vi "quote and escape json string 2.vi"(11 "base string":string) -> (3 "String out":string)   [LabVIEW 2020, in "JSONtext.lvlib"]
uses:
  <vilib>/JDP Science/JSONtext/JSONtext.lvlib
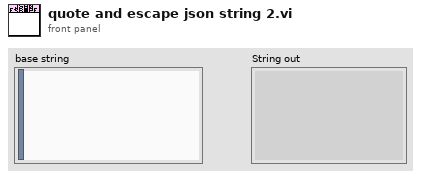
[diagram p1: front panel]
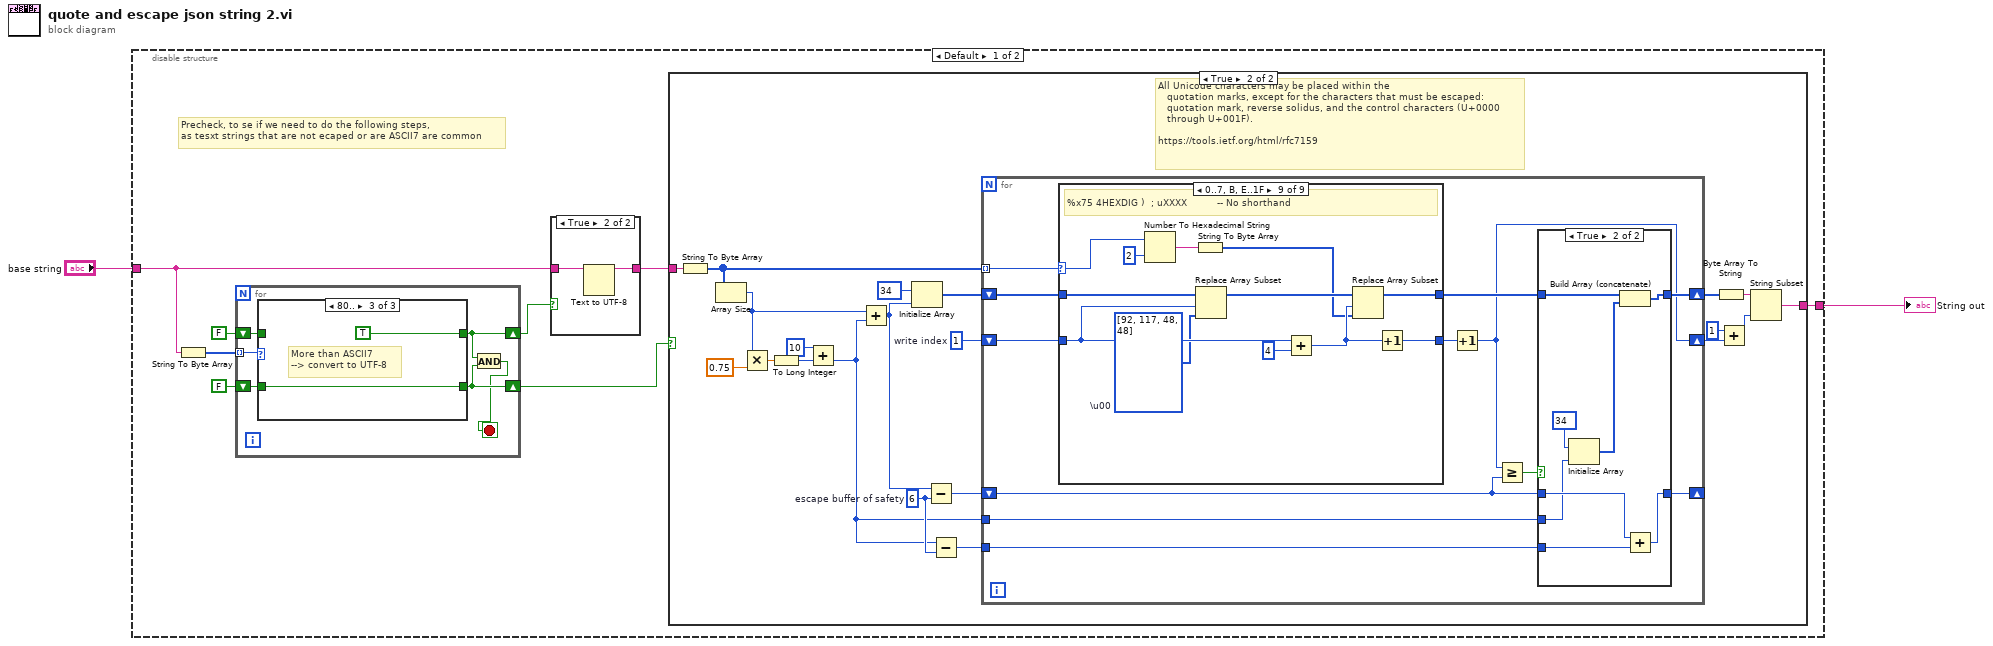
[diagram p0: block diagram]
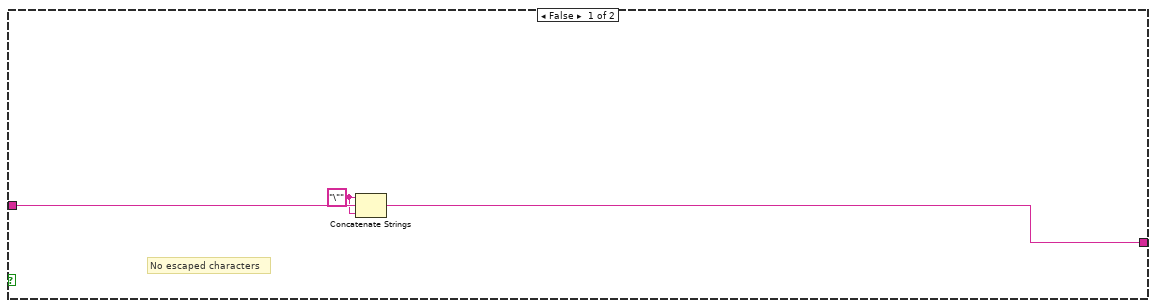
[diagram p2: hidden frame]
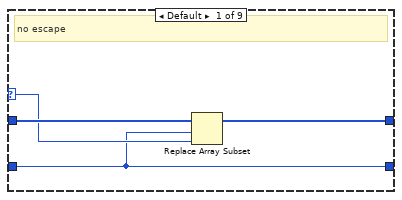
[diagram p4: hidden frame]
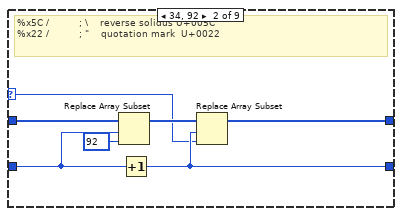
[diagram p5: hidden frame]
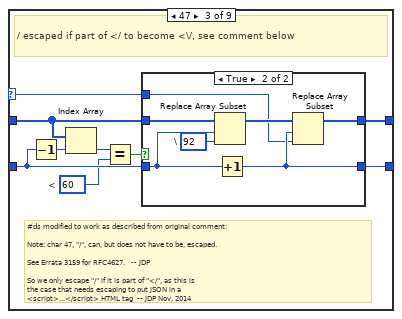
[diagram p6: hidden frame]
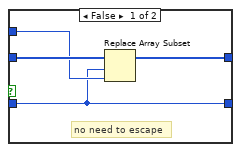
[diagram p7: hidden frame]
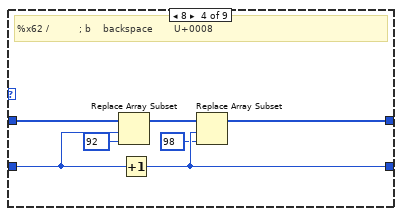
[diagram p8: hidden frame]
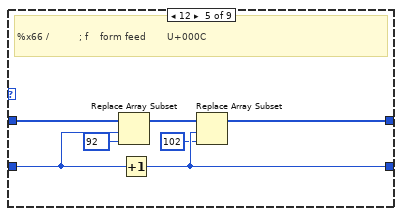
[diagram p9: hidden frame]
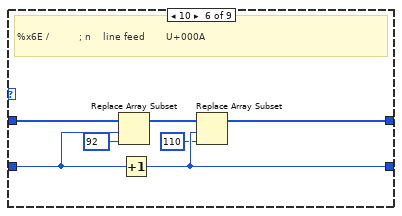
[diagram p10: hidden frame]
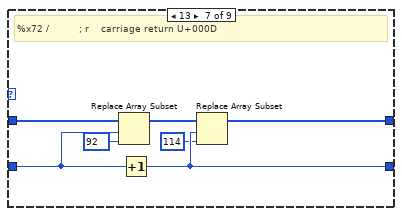
[diagram p11: hidden frame]
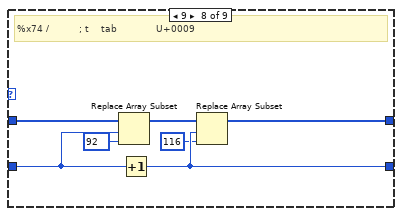
[diagram p12: hidden frame]
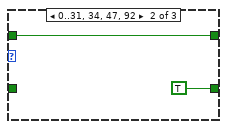
[diagram p15: hidden frame]
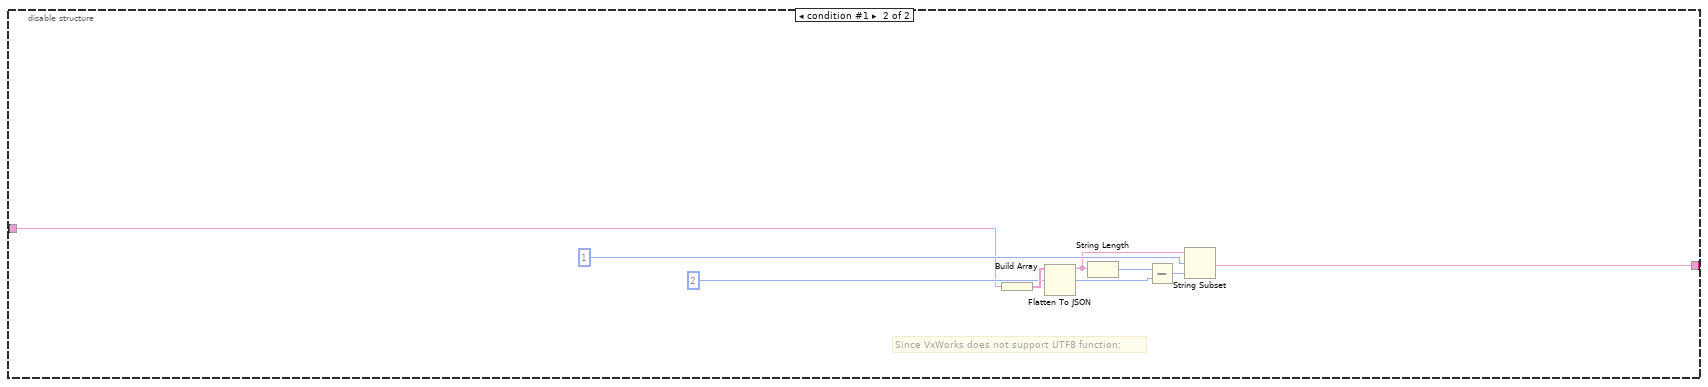
[diagram p16: hidden frame]
diagram:
  n1 = disable-structure shown="Default" {
    disable-tunnel: [w10 w151] -> w2
    disable-tunnel: "base string" -> [w8 w150]
    frame condition #0 (active) {
      # "Precheck, to se if we need to do the following steps,\nas tesxt strings that are not ecaped or are ASCII7 are common"
      n2 = String To Byte Array(string=w8) -> (unsigned byte array=w7:u8[])
      n3 = for {
        tunnel: w7 -> [w143] mode=indexing
        shift-right: [w142] -> w4
        shift-left: FALSE -> [w139]
        shift-right: [w141] -> w3
        shift-left: FALSE -> [w138]
        stop <- w140 stop-if-true
        n4 = case shown="80.." w143 {
          tunnel: [w145 w146 TRUE] -> w142
          tunnel: [w144 TRUE w148] -> w141
          tunnel: w139 -> [w145 w146 _]
          tunnel: w138 -> [w144 _ w148]
          frame Default {
          }
          frame 0..31, 34, 47, 92 {
          }
          frame 128.. {
            # "More than ASCII7\n--> convert to UTF-8"
          }
        }
        n5 = And(x=w142, y=w141) -> (x .and. y?=w140:bool)
      }
      n6 = case shown="True" w4 {
        tunnel: [w135 w137] -> w9
        tunnel: w8 -> [w135 w136]
        frame False {
        }
        frame True {
          n7 = Text to UTF-8(11:w136) -> (3:w137:string)  [unwired: 2 in, 1 out]
        }
      }
      n8 = case shown="True" w3 {
        tunnel: [w12 w34] -> w10
        tunnel: w9 -> [w13 w14]
        frame False {
          w11 = "\"" ("string")
          # "No escaped characters"
          n9 = Concatenate Strings(w11, w13, w11) -> (w12:string)
        }
        frame True {
          w20 = 6  # escape buffer of safety
          w32 = 1  # write index
          # "All Unicode characters may be placed within the\n   quotation marks, except for the characters that must be escaped:\n   quotation mark, reverse solidus, and the control characters (U+0000\n   through U+001F).\n\nhttps://tools.ietf.org/html/rfc7159"
          n10 = String To Byte Array(string=w14) -> (unsigned byte array=w26:u8[])
          n11 = Array Size(array=w26) -> (size(s)=w24:i32)
          n12 = Multiply(x=w24, y=0.75) -> (x*y=w27:dbl)
          n13 = To Long Integer(number=w27) -> (32bit integer=w21:i32)
          n14 = Add(x=10, y=w21) -> (x+y=w17:i32)
          n15 = Add(x=w24, y=w17) -> (x+y=w23:i32)
          n16 = Initialize Array(u8 34, w23) -> (w29:u8[])
          n17 = Subtract(x=w23, y=w20) -> (x-y=w22:i32)
          n18 = Subtract(x=w17, y=w20) -> (x-y=w19:i32)
          n19 = for {
            shift-right: [w43] -> w31
            shift-left: w29 -> [w46]
            shift-right: [w36] -> w25
            shift-left: w32 -> [w45]
            tunnel: w26 -> [w44] mode=indexing
            shift-right: [w40] -> _
            shift-left: w22 -> [w39]
            tunnel: w17 -> [w38]
            tunnel: w19 -> [w37]
            n20 = case shown="0..7, B, E..1F" w44 {
              selector: w44 -> [w58 w62 w74 _ _ _ _ _ w131]
              tunnel: w46 -> [w60 w67 w73 w94 w101 w108 w115 w122 w134]
              tunnel: [w59 w64 w76 w91 w98 w105 w112 w119 w133] -> w42
              tunnel: w45 -> [w57 w65 w72 w92 w99 w106 w113 w120 w132]
              tunnel: [w57 w63 w75 w90 w97 w104 w111 w118 w123] -> w41
              frame Default {
                # "no escape"
                n21 = Replace Array Subset(array=w60, new element=w58, index=w57) -> (w59:u8[])
              }
              frame 34, 92 {
                # "%x5C /          ; \\    reverse solidus U+005C\n%x22 /          ; \"    quotation mark  U+0022"
                n22 = Replace Array Subset(array=w67, new element=u8 92 ("new element/subarray"), index=w65) -> (w66:u8[])
                n23 = Increment(x=w65) -> (x+1=w63:i32)
                n24 = Replace Array Subset(array=w66, new element=w62, index=w63) -> (w64:u8[])
              }
              frame 47 {
                w68 = u8 60  # <
                # "#ds modified to work as described from original comment:\n\nNote: char 47, \"/\", can, but does not have to be, escaped.\n\nSee Errata 3159 for RFC4627.   -- JDP\n\nSo we only escape \"/\" if it is part of \"</\", as this is\nthe case that needs escaping to put JSON in a\n<script>...</script> HTML tag  -- JDP Nov, 2014"
                # "/ escaped if part of </ to become <\\/, see comment below"
                n25 = Decrement(x=w72) -> (x-1=w71:i32)
                n26 = Index Array(array=w73, index=w71) -> (element=w70:u8)
                n27 = Equal?(x=w70, y=w68) -> (x = y?=w69:bool)
                n28 = case shown="True" w69 {
                  tunnel: [w79 w86] -> w76
                  tunnel: [w77 w85] -> w75
                  tunnel: w74 -> [w78 w84]
                  tunnel: w73 -> [w80 w83]
                  tunnel: w72 -> [w77 w82]
                  frame False {
                    # "no need to escape"
                    n29 = Replace Array Subset(array=w80, new element=w78, index=w77) -> (w79:u8[])
                  }
                  frame True {
                    w81 = u8 92  # \
                    n30 = Replace Array Subset(array=w83, new element=w81, index=w82) -> (w87:u8[])
                    n31 = Increment(x=w82) -> (x+1=w85:i32)
                    n32 = Replace Array Subset(array=w87, new element=w84, index=w85) -> (w86:u8[])
                  }
                }
              }
              frame 8 {
                # "%x62 /          ; b    backspace       U+0008"
                n33 = Replace Array Subset(array=w94, new element=u8 92 ("new element/subarray"), index=w92) -> (w93:u8[])
                n34 = Increment(x=w92) -> (x+1=w90:i32)
                n35 = Replace Array Subset(array=w93, new element=u8 98 ("new element/subarray"), index=w90) -> (w91:u8[])
              }
              frame 12 {
                # "%x66 /          ; f    form feed       U+000C"
                n36 = Replace Array Subset(array=w101, new element=u8 92 ("new element/subarray"), index=w99) -> (w100:u8[])
                n37 = Increment(x=w99) -> (x+1=w97:i32)
                n38 = Replace Array Subset(array=w100, new element=u8 102 ("new element/subarray"), index=w97) -> (w98:u8[])
              }
              frame 10 {
                # "%x6E /          ; n    line feed       U+000A"
                n39 = Replace Array Subset(array=w108, new element=u8 92 ("new element/subarray"), index=w106) -> (w107:u8[])
                n40 = Increment(x=w106) -> (x+1=w104:i32)
                n41 = Replace Array Subset(array=w107, new element=u8 110 ("new element/subarray"), index=w104) -> (w105:u8[])
              }
              frame 13 {
                # "%x72 /          ; r    carriage return U+000D"
                n42 = Replace Array Subset(array=w115, new element=u8 92 ("new element/subarray"), index=w113) -> (w114:u8[])
                n43 = Increment(x=w113) -> (x+1=w111:i32)
                n44 = Replace Array Subset(array=w114, new element=u8 114 ("new element/subarray"), index=w111) -> (w112:u8[])
              }
              frame 9 {
                # "%x74 /          ; t    tab             U+0009"
                n45 = Replace Array Subset(array=w122, new element=u8 92 ("new element/subarray"), index=w120) -> (w121:u8[])
                n46 = Increment(x=w120) -> (x+1=w118:i32)
                n47 = Replace Array Subset(array=w121, new element=u8 116 ("new element/subarray"), index=w118) -> (w119:u8[])
              }
              frame 0..7, 11, 14..31 {
                w124 = u8[] [92, 117, 48, 48]  # \u00
                # "%x75 4HEXDIG )  ; uXXXX          -- No shorthand"
                n48 = Number To Hexadecimal String(1:i16 2 ("width (-)"), 2:w131) -> (0:w126:string)
                n49 = String To Byte Array(string=w126) -> (unsigned byte array=w128:u8[])
                n50 = Replace Array Subset(array=w134, new element=w124, index=w132) -> (w130:u8[])
                n51 = Add(x=w132, y=4) -> (x+y=w129:i32)
                n52 = Replace Array Subset(array=w130, new element=w128, index=w129) -> (w133:u8[])
                n53 = Increment(x=w129) -> (x+1=w123:i32)
              }
            }
            n54 = Increment(x=w41) -> (x+1=w36:i32)
            n55 = Greater Or Equal?(x=w36, y=w39) -> (x >= y?=w35:bool)
            n56 = case shown="True" w35 {
              tunnel: [w48 w51] -> w43
              tunnel: w42 -> [w48 w52]
              tunnel: [w47 w54] -> w40
              tunnel: w39 -> [w47 w55]
              tunnel: w38 -> [_ w53]
              tunnel: w37 -> [_ w56]
              frame False {
              }
              frame True {
                n57 = Initialize Array(u8 34, w53) -> (w50:u8[])
                n58 = Build Array (concatenate)(w52, w50) -> (w51:u8[])
                n59 = Add(x=w55, y=w56) -> (x+y=w54:i32)
              }
            }
          }
          n60 = Byte Array To String(unsigned byte array=w31) -> (string=w33:string)
          n61 = Add(x=1, y=w25) -> (x+y=w18:i32)
          n62 = String Subset(string=w33, length (rest)=w18) -> (substring=w34:string)  [unwired: 1 in]
        }
      }
    }
    frame condition #1 {
      # "Since VxWorks does not support UTF8 function:"
      n63 = Build Array(w150) -> (w157:string[])
      n64 = Flatten To JSON(anything=w157) -> (JSON string=w154:string)  [unwired: 2 in, 1 out]
      n65 = String Length(string=w154) -> (length=w155:i32)
      n66 = Subtract(x=w155, y=2 ("x")) -> (x-y=w153:i32)
      n67 = String Subset(string=w154, offset (0)=1, length (rest)=w153) -> (substring=w151:string)
    }
  }
  "String out" <- w2
